vi "Ball Screw Control.vi"(4 "FeederButton":bool, 5 "Target Button":bool, 6 "PyramidButton":bool, 7 "Joystick Axis":dbl, 8 "Bottom Limit":bool, 9 "Top Limit":bool, 10 "Closed Loop On/Off":bool, 11 "Ball Screw DevRef In":T1={"DeviceStatus"={"status"=FALSE, "code"=0, "source"=""}, "Type"=enum."PWM", "PWM"={"Digital Module"=enum."Digital Module 1", "PWM Channel"=enum."Invalid", "DeadBand"={"Name"="", "maxPositivePwm"=0, "minPositivePwm"=0, "centerPwm"=0, "maxNegativePwm"=0, "minNegativePwm"=0, "angularRange"=0}}, "CAN"={"Device Number"=0, "Control Mode"=enum."Percent VBus", "Semaphore"=refnum, "Max Vout"=12.0}, "Invert"=FALSE, "TransformRef"=refnum, "InvTransformRef"=refnum}) -> (2 "Motor Output":dbl, 3 "Ball Screw DevRef Out":T1={"DeviceStatus"={"status"=FALSE, "code"=0, "source"=""}, "Type"=enum."PWM", "PWM"={"Digital Module"=enum."Digital Module 1", "PWM Channel"=enum."Invalid", "DeadBand"={"Name"="", "maxPositivePwm"=0, "minPositivePwm"=0, "centerPwm"=0, "maxNegativePwm"=0, "minNegativePwm"=0, "angularRange"=0}}, "CAN"={"Device Number"=0, "Control Mode"=enum."Percent VBus", "Semaphore"=refnum, "Max Vout"=12.0}, "Invert"=FALSE, "TransformRef"=refnum, "InvTransformRef"=refnum})   [LabVIEW 2012]
uses:
  <vilib>/Rock Robotics/WPI/MotorControl/WPI_MotorControlDeviceRef.ctl
  <vilib>/Rock Robotics/SystemInterfaces/Typedef/FPGA_TypedefDigitalModule.ctl
  <vilib>/Rock Robotics/SystemInterfaces/DIO/FPGA_DIOPWMChannel.ctl
  <vilib>/Rock Robotics/WPI/PWM/WPI_PWMDeadband.ctl
  <vilib>/Rock Robotics/WPI/CAN/Jaguar/SubVIs/WPI_CANJaguar_ControlMode.ctl
  <vilib>/Rock Robotics/WPI/PWM/WPI_PWMTransform_ConPane.ctl
  <vilib>/Rock Robotics/WPI/DriverStation/DriverStationLCD/WPI_DriverStationLCDLCDLine.ctl
  <vilib>/Rock Robotics/WPI/CAN/Jaguar/SubVIs/WPI_CANJaguar_PositionReference.ctl
  Robot Global Data.vi
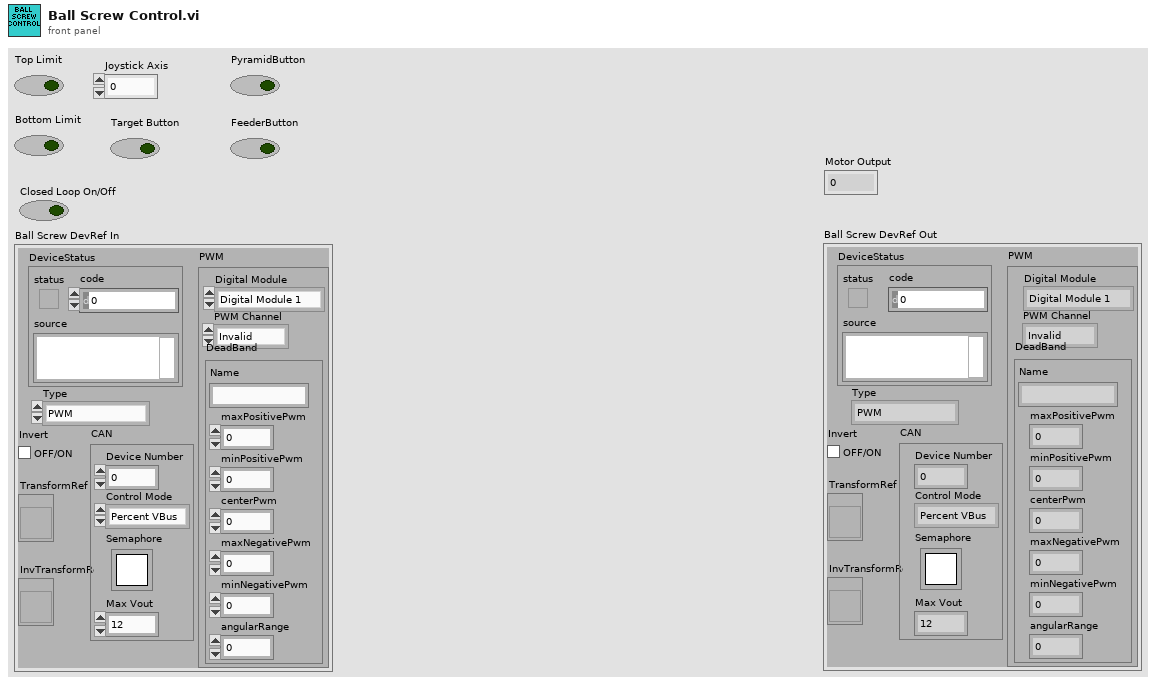
[diagram p1: front panel]
types:
  T1 = typedef "WPI_MotorControlDeviceRef.ctl" = cluster{"DeviceStatus":errorcluster, "Type":enum16{"PWM", "CAN"}, "PWM":cluster{"Digital Module":T2, "PWM Channel":T3, "DeadBand":T4}, "CAN":cluster{"Device Number":u8, "Control Mode":T5, "Semaphore":T6, "Max Vout":dbl}, "Invert":bool, "TransformRef":T7, "InvTransformRef":T7}
  T2 = typedef "FPGA_TypedefDigitalModule.ctl" = enum16{"Digital Module 1", "Digital Module 2"}
  T3 = typedef "FPGA_DIOPWMChannel.ctl" = enum8{"PWM 1", "PWM 2", "PWM 3", "PWM 4", "PWM 5", "PWM 6", "PWM 7", "PWM 8", "PWM 9", "PWM 10", "Invalid"}
  T4 = typedef "WPI_PWMDeadband.ctl" = cluster{"Name":string, "maxPositivePwm":i32, "minPositivePwm":i32, "centerPwm":i32, "maxNegativePwm":i32, "minNegativePwm":i32, "angularRange":u16}
  T5 = typedef "WPI_CANJaguar_ControlMode.ctl" = enum8{"Percent VBus", "Current", "Speed", "Position", "Voltage"}
  T6 = typedef "Semaphore RefNum" = refnum<k1>
  T7 = typedef "WPI_PWMTransform_ConPane.ctl" = refnum<vi>
  T8 = typedef "WPI_DriverStationLCDLCDLine.ctl" = enum16{"Main - Line 1", "User - Line 2", "User - Line 3", "User - Line 4", "User - Line 5", "User - Line 6"}
  T9 = typedef "WPI_CANJaguar_PositionReference.ctl" = u8
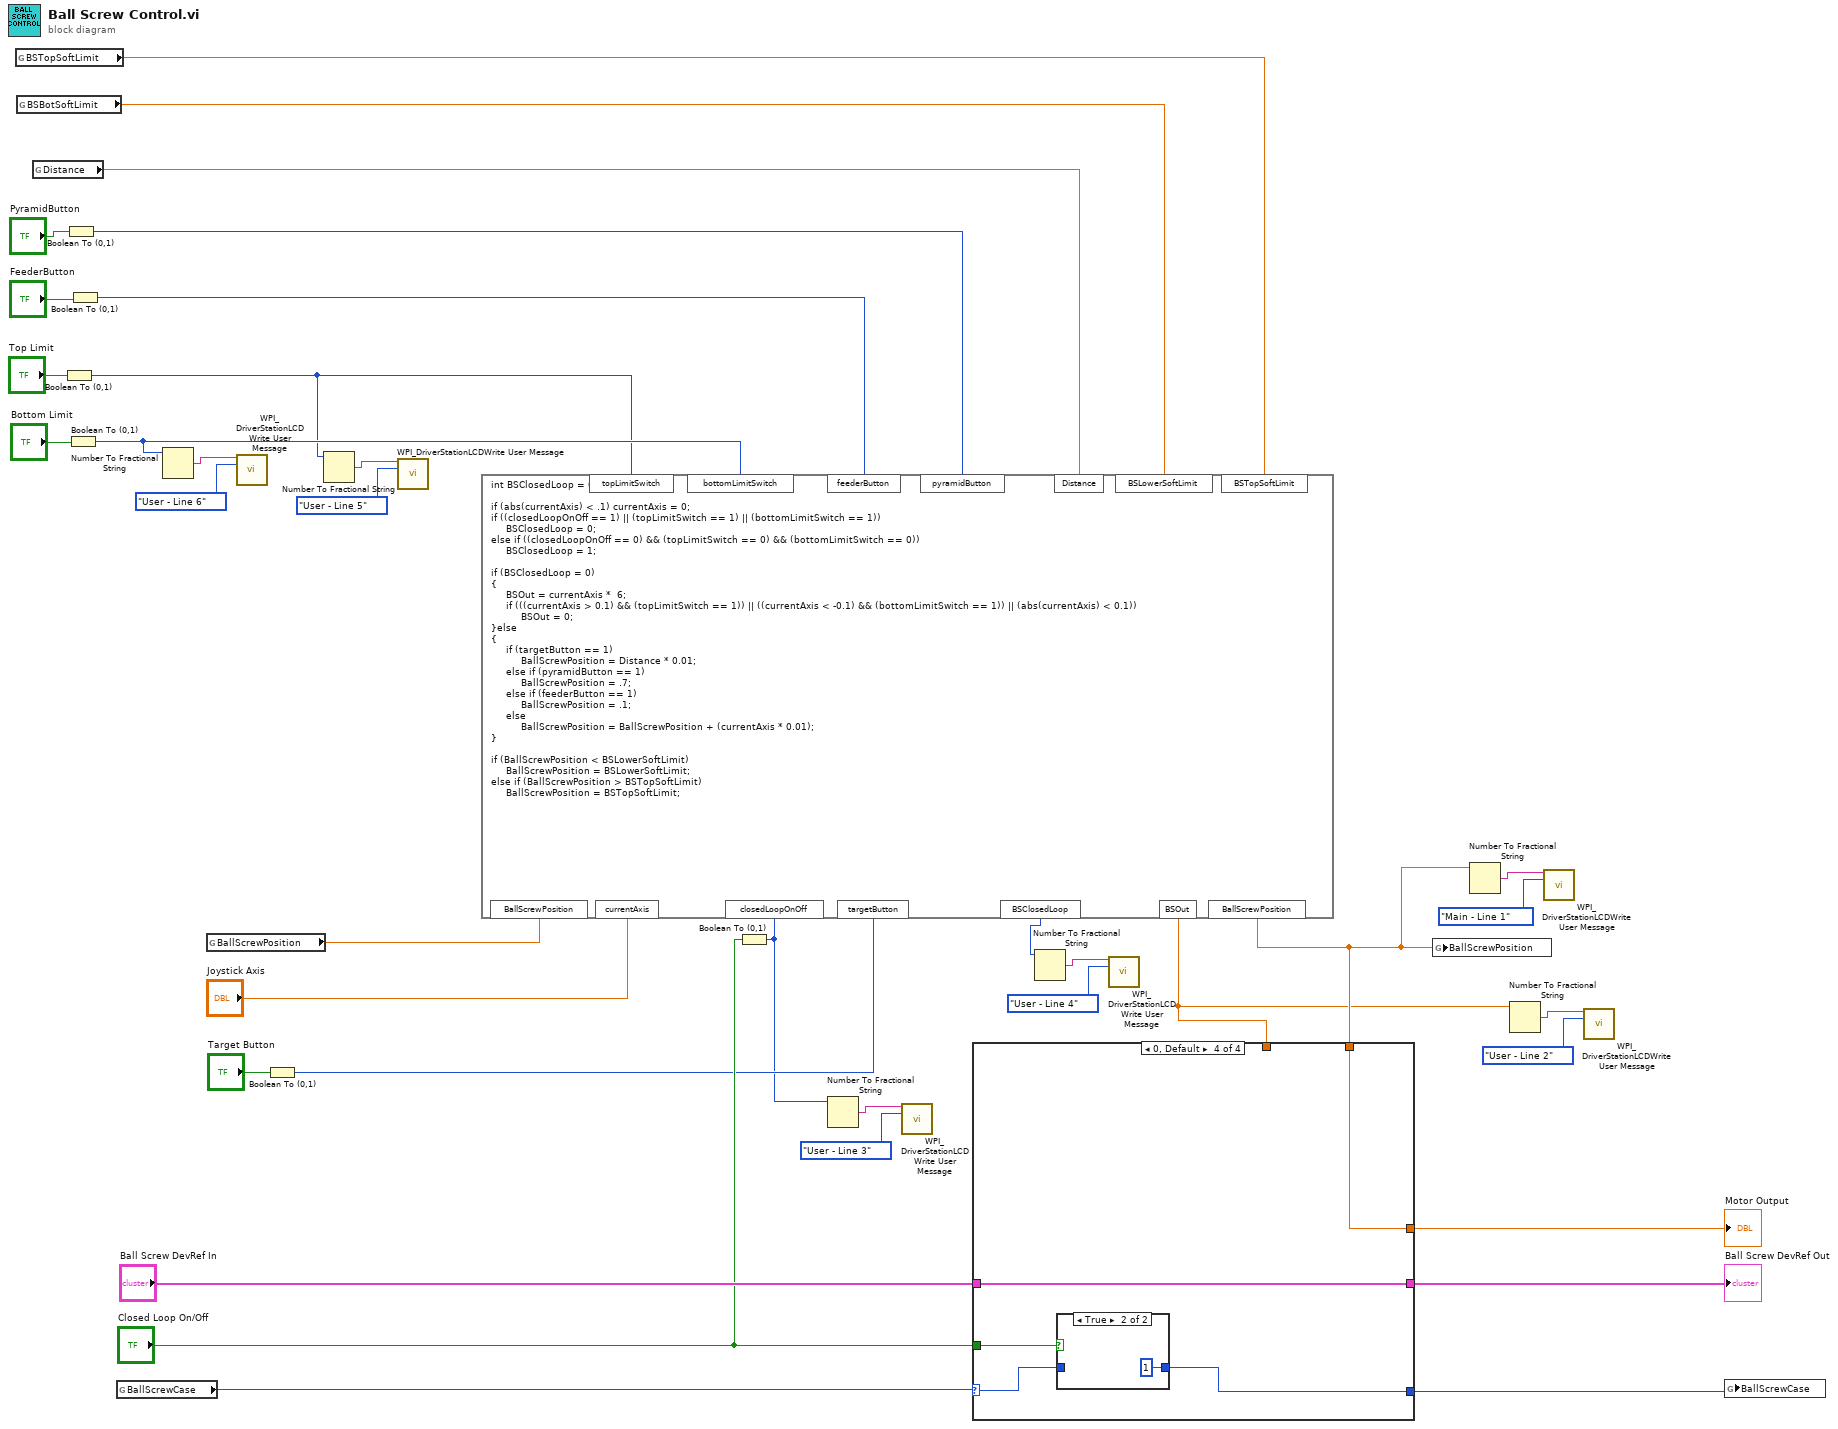
[diagram p0: block diagram]
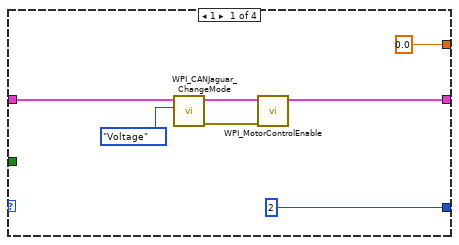
[diagram p2: hidden frame]
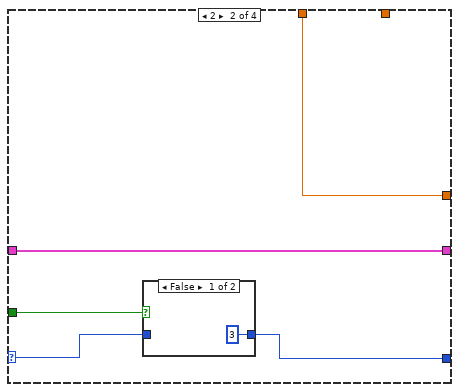
[diagram p3: hidden frame]
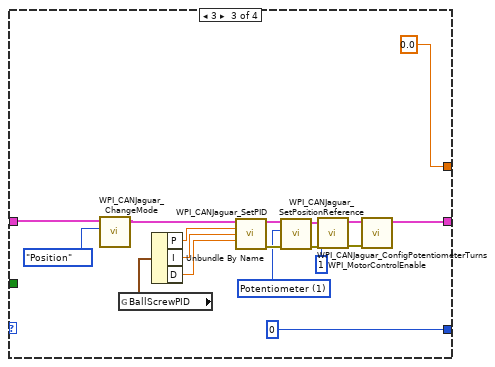
[diagram p5: hidden frame]
diagram:
  n1 = global read "Robot Global Data.vi" "BSTopSoftLimit"() -> (w27:dbl)
  n2 = global read "Robot Global Data.vi" "BSBotSoftLimit"() -> (w26:dbl)
  n3 = global read "Robot Global Data.vi" "Distance"() -> (w28:dbl)
  n4 = Boolean To (0,1)(Boolean="Top Limit") -> (0, 1=w11:i16)
  n5 = Boolean To (0,1)(Boolean="PyramidButton") -> (0, 1=w20:i16)
  n6 = Boolean To (0,1)(Boolean="Bottom Limit") -> (0, 1=w14:i16)
  n7 = Boolean To (0,1)(Boolean="FeederButton") -> (0, 1=w22:i16)
  n8 = global read "Robot Global Data.vi" "BallScrewCase"() -> (w37:i8)
  n9 = Number To Fractional String(number=w14) -> (F-format string=w16:string)  [unwired: 3 in]
  n10 = global read "Robot Global Data.vi" "BallScrewPosition"() -> (w29:dbl)
  n11 = call <vilib>:"WPI_DriverStationLCDWrite User Message.vi"("line text"=w16, "line"=WPI_DriverStationLCDLCDLine."User - Line 6") -> ()  [unwired: 13 in, 1 out]
  n12 = Boolean To (0,1)(Boolean="Target Button") -> (0, 1=w30:i16)
  n13 = Number To Fractional String(number=w11) -> (F-format string=w13:string)  [unwired: 3 in]
  n14 = call <vilib>:"WPI_DriverStationLCDWrite User Message.vi"("line text"=w13, "line"=WPI_DriverStationLCDLCDLine."User - Line 5") -> ()  [unwired: 13 in, 1 out]
  n15 = Boolean To (0,1)(Boolean="Closed Loop On/Off") -> (0, 1=w1:i16)
  n16 = formula code="int BSClosedLoop = 0;\n\nif (abs(currentAxis) < .1) currentAxis = 0;\nif ((closedLoopOnOff == 1) || (topLimitSwitch == 1) || (bottomLimitSwitch == 1))\n     BSClosedLoop = 0;\nelse if ((closedLoopOnOff == 0) && (topLimitSwitch == 0) && (bottomLimitSwitch == 0))\n     BSClosedLoop = 1;\n\nif (BSClosedLoop = 0)\n{\n     BSOut = currentAxis *  6;\n     if (((currentAxis > 0.1) && (topLimitSwitch == 1)) || ((currentAxis < -0.1) && (bottomLimitSwitch == 1)) || (abs(currentAxis) < 0.1))\n          BSOut = 0;\n}else\n{\n     if (targetButton == 1)\n          BallScrewPosition = Distance * 0.01;\n     else if (pyramidButton == 1)\n          BallScrewPosition = .7;\n     else if (feederButton == 1)\n          BallScrewPosition = .1;\n     else\n          BallScrewPosition = BallScrewPosition + (currentAxis * 0.01);\n}\n\nif (BallScrewPosition < BSLowerSoftLimit)\n     BallScrewPosition = BSLowerSoftLimit;\nelse if (BallScrewPosition > BSTopSoftLimit)\n     BallScrewPosition = BSTopSoftLimit;"("closedLoopOnOff"=w1, "topLimitSwitch"=w11, "bottomLimitSwitch"=w14, "BallScrewPosition"=w29, "currentAxis"="Joystick Axis", "targetButton"=w30, "Distance"=w28, "BSLowerSoftLimit"=w26, "BSTopSoftLimit"=w27, "pyramidButton"=w20, "feederButton"=w22) -> ("BSOut"=w8:dbl, "BallScrewPosition"=w17:dbl, "BSClosedLoop"=w4:i32)
  n17 = Number To Fractional String(number=w1) -> (F-format string=w3:string)  [unwired: 3 in]
  n18 = call <vilib>:"WPI_DriverStationLCDWrite User Message.vi"("line text"=w3, "line"=WPI_DriverStationLCDLCDLine."User - Line 3") -> ()  [unwired: 13 in, 1 out]
  n19 = case shown="0, Default" w37 {
    selector: w37 -> [_ w47 _ w71]
    tunnel: [i8 2 ("ShooterCase") w46 i8 0 ("ShooterCase") w72] -> w7
    tunnel: "Ball Screw DevRef In" -> [w43 w49 w68 w74]
    tunnel: [w39 w49 w55 w74] -> w24
    tunnel: "Closed Loop On/Off" -> [_ w48 _ w73]
    tunnel: [0.0 ("FSpeed") w45 0.0 ("FSpeed") w70] -> w25
    tunnel: w8 -> [_ w45 _ _]
    tunnel: w17 -> [_ _ _ w70]
    frame 1 {
      n20 = call <vilib>:"WPI_CANJaguar_ChangeMode.vi"("Control Mode"=WPI_CANJaguar_ControlMode."Voltage", "CAN Jaguar Ref"=w43) -> ("error out"=w40:errorcluster, "CAN Jaguar Ref Out"=w41:T1)  [unwired: 8 in]
      n21 = call <vilib>:"WPI_MotorControlEnable.vi"("error in (no error)"=w40, "CAN Jaguar Ref"=w41) -> ("CAN Jaguar Ref Out"=w39:T1)  [unwired: 8 in, 1 out]
    }
    frame 2 {
      n22 = case shown="False" w48 {
        tunnel: [i8 3 ("ShooterCase") w51] -> w46
        tunnel: w47 -> [_ w51]
        frame False {
        }
        frame True {
        }
      }
    }
    frame 3 {
      w53 = T9 1 items=["Quad Encoder"=0, "Potentiometer"=1, "None"=255] ("Position Reference")
      n23 = call <vilib>:"WPI_CANJaguar_ChangeMode.vi"("Control Mode"=WPI_CANJaguar_ControlMode."Position", "CAN Jaguar Ref"=w68) -> ("CAN Jaguar Ref Out"=w63:T1)  [unwired: 8 in, 1 out]
      n24 = global read "Robot Global Data.vi" "BallScrewPID"() -> (w67:cluster{"P":dbl, "I":dbl, "D":dbl})
      n25 = Unbundle By Name(w67) -> ("P"=w66:dbl, "I"=w65:dbl, "D"=w64:dbl)
      n26 = call <vilib>:"WPI_CANJaguar_SetPID.vi"("CAN Jaguar Ref"=w63, "P"=w66, "I"=w65, "D"=w64) -> ("CAN Jaguar Ref Out"=w61:T1, "error out"=w60:errorcluster)  [unwired: 10 in]
      n27 = call <vilib>:"WPI_CANJaguar_SetPositionReference.vi"("error in (no error)"=w60, "Position Reference"=w53, "CAN Jaguar Ref"=w61) -> ("error out"=w58:errorcluster, "CAN Jaguar Ref Out"=w59:T1)  [unwired: 7 in]
      n28 = call <vilib>:"WPI_CANJaguar_ConfigPotentiometerTurns.vi"("error in (no error)"=w58, "Potentiometer Turns"=u16 1, "CAN Jaguar Ref"=w59) -> ("error out"=w57:errorcluster, "CAN Jaguar Ref Out"=w56:T1)  [unwired: 7 in]
      n29 = call <vilib>:"WPI_MotorControlEnable.vi"("error in (no error)"=w57, "CAN Jaguar Ref"=w56) -> ("CAN Jaguar Ref Out"=w55:T1)  [unwired: 8 in, 1 out]
    }
    frame 0, Default {
      n30 = case shown="True" w73 {
        tunnel: [w75 i8 1 ("ShooterCase")] -> w72
        tunnel: w71 -> [w75 _]
        frame False {
        }
        frame True {
        }
      }
    }
  }
  "Motor Output" <- w25
  "Ball Screw DevRef Out" <- w24
  n31 = Number To Fractional String(number=w4) -> (F-format string=w6:string)  [unwired: 3 in]
  n32 = call <vilib>:"WPI_DriverStationLCDWrite User Message.vi"("line text"=w6, "line"=WPI_DriverStationLCDLCDLine."User - Line 4") -> ()  [unwired: 13 in, 1 out]
  n33 = global write "Robot Global Data.vi" "BallScrewPosition"(w17) -> ()
  n34 = Number To Fractional String(number=w17) -> (F-format string=w19:string)  [unwired: 3 in]
  n35 = Number To Fractional String(number=w8) -> (F-format string=w10:string)  [unwired: 3 in]
  n36 = call <vilib>:"WPI_DriverStationLCDWrite User Message.vi"("line text"=w19, "line"=WPI_DriverStationLCDLCDLine."Main - Line 1") -> ()  [unwired: 13 in, 1 out]
  n37 = call <vilib>:"WPI_DriverStationLCDWrite User Message.vi"("line text"=w10, "line"=WPI_DriverStationLCDLCDLine."User - Line 2") -> ()  [unwired: 13 in, 1 out]
  n38 = global write "Robot Global Data.vi" "BallScrewCase"(w7) -> ()
